vi "Open CANOpen Session.vi"(8 "error in (no error)":errorcluster) -> (0 "error out":errorcluster, 3 "interface object out":refnum<k20>)   [LabVIEW 2016]
uses:
  Motor controllers.vi
  <vilib>/CANopenLib/CANOPEN.llb/CANopen Interface Create.vi
  Settings.lvlib
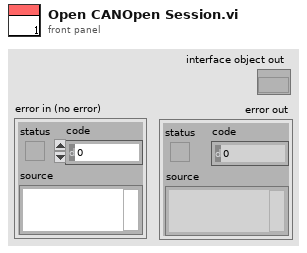
[diagram p1: front panel]
types:
  T1 = cluster{"termination resistor":bool, "CANopen interface":u32, "baud rate":u32, "FPGA VI Reference":refnum<k20>, "interface object out":refnum<k20>}
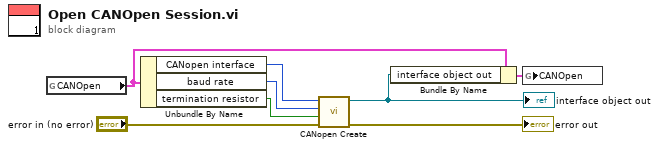
[diagram p0: block diagram]
diagram:
  n1 = global read "Motor controllers.vi" "CANOpen"() -> (w4:T1)
  n2 = Unbundle By Name(w4) -> ("CANopen interface"=w8:u32, "baud rate"=w7:u32, "termination resistor"=w6:bool)
  n3 = call-poly <vilib>:"CANopen Create.vi"("error in (no error)"="error in (no error)", "termination? (F)"=w6, "baud rate"=w7, "interface name"=w8) -> ("error out"=→"error out":errorcluster, "interface object out"=w5:refnum<k20>)  [unwired: 6 in]
  "interface object out" <- w5
  n4 = Bundle By Name(cluster=w4, "interface object out"=w5) -> (w3:T1)
  n5 = global write "Motor controllers.vi" "CANOpen"(w3) -> ()
